vi "Test.vi"   [LabVIEW 2019]
doc: "This VI is called when test mode begins, and will automatically be terminated when it ends. You can add manual or automatic tests and invoke them from the dashboard."
uses:
  Globals/Joystick_Globals.vi
types:
  T1 = typedef "Joystick_Controls.ctl" = cluster{"Pilot Left Joystick X":dbl, "Pilot Left Joystick Y":dbl, "Pilot A Button":bool, "Pilot B Button":bool, "Pilot X Button":bool, "Pilot Y Button":bool, "Pilot Left Bumper":bool, "Pilot Right Bumper":bool, "Pilot View Button":bool, "Pilot Menu Button":bool, "Pilot Left Joystick Press":bool, "Pilot Right Joystick Press":bool, "Pilot Left Trigger":dbl, "Pilot Right Joystick X":dbl, "Pilot Right Joystick Y":dbl, "Pilot Right Trigger":dbl, "Copilot Left Joystick X":dbl, "Copilot Left Joystick Y":dbl, "Copilot A Button":bool, "Copilot B Button":bool, "Copilot X Button":bool, "Copilot Y Button":bool, "Copilot Left Bumper":bool, "Copilot Right Bumper":bool, "Copilot View Button":bool, "Copilot Menu Button":bool, "Copilot Left Joystick Press":bool, "Copilot Right Joystick Press":bool, "Copilot Left Trigger":dbl, "Copilot Right Joystick X":dbl, "Copilot Right Joystick Y":dbl, "Copilot Right Trigger":dbl, "Pilot D-pad North":bool, "Pilot D-pad South":bool, "Pilot D-pad East":bool, "Pilot D-pad West":bool, "Pilot D-pad NE ":bool, "Pilot D-pad SE":bool, "Pilot D-pad SW":bool, "Pilot D-pad NW":bool, "CoPilot D-pad North":bool, "CoPilot D-pad South":bool, "CoPilot D-pad East":bool, "CoPilot D-pad West":bool, "CoPilot D-pad NE":bool, "CoPilot D-pad SE":bool, "CoPilot D-pad SW":bool, "CoPilot D-pad NW":bool, "Pilot Left Trigger Pressed":bool, "Pilot Right Trigger Pressed":bool, "CoPilot Left Trigger Pressed":bool, "CoPilot Right Trigger Pressed":bool}
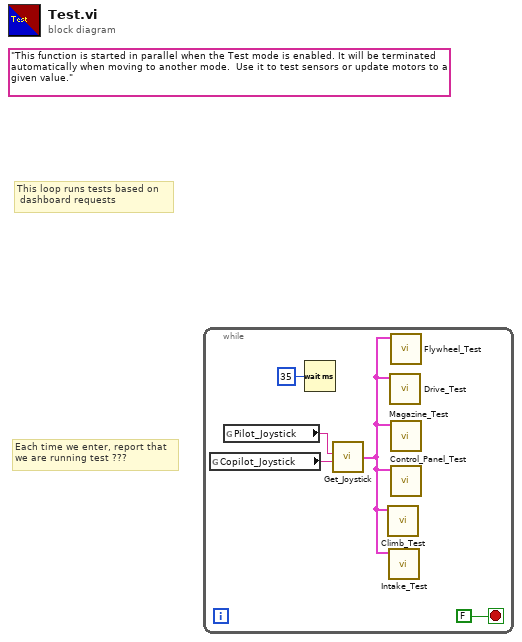
[diagram p0: block diagram]
diagram:
  (unwired) "This function is started in parallel when the Test mode is enabled. It will be terminated automatically when moving to another mode.  Use it to test sensors or update motors to a given value."
  # "This loop runs tests based on \n dashboard requests"
  # "Each time we enter, report that\nwe are running test ???"
  n1 = while {
    stop <- FALSE stop-if-true
    n2 = global read "Joystick_Globals.vi" "Copilot_Joystick"() -> (w4:string)
    n3 = global read "Joystick_Globals.vi" "Pilot_Joystick"() -> (w5:string)
    n4 = Wait (ms)(milliseconds to wait=u32 35) -> ()  [unwired: 1 out]
    n5 = call "Get_Joystick.vi"("Joystick_One"=w5, "Joystick_Two"=w4) -> ("Joystick_Out"=w1:T1)  [unwired: 5 in]
    n6 = call "Climb_Test.vi"("Joystick_In"=w1) -> ()  [unwired: 11 in]
    n7 = call "Intake_Test.vi"("Joystick_In"=w1) -> ()  [unwired: 11 in]
    n8 = call "Drive_Test.vi"("Joystick_In"=w1) -> ()  [unwired: 11 in]
    n9 = call "Flywheel_Test.vi"("Joystick_IN"=w1) -> ()  [unwired: 11 in]
    n10 = call "Magazine_Test.vi"("Joystick_In"=w1) -> ()  [unwired: 11 in]
    n11 = call "Control_Panel_Test.vi"("Joystick_In"=w1) -> ()  [unwired: 11 in]
  }
